vi "Open.vi"(8 "error in (no error)":errorcluster, 11 "MelsecTCP in":refnum<class "InovanceSerialModbusRtu.lvclass">) -> (0 "error out":errorcluster, 3 "MelsecTCP out":refnum<class "InovanceSerialModbusRtu.lvclass">)   [LabVIEW 2020, in "HslCommunication.lvlib" / "InovanceSerialModbusRtu.lvclass"]
uses:
  InovanceSerialModbusRtu.lvclass
  InovanceSerialModbusRtu.lvclass/InovanceSerialModbusRtu.ctl
  E:/Git/Libraries/develop/HslCommunication/_Dependenciecs/HslCommunication.dll
  _Dependenciecs/HslCommunication.dll
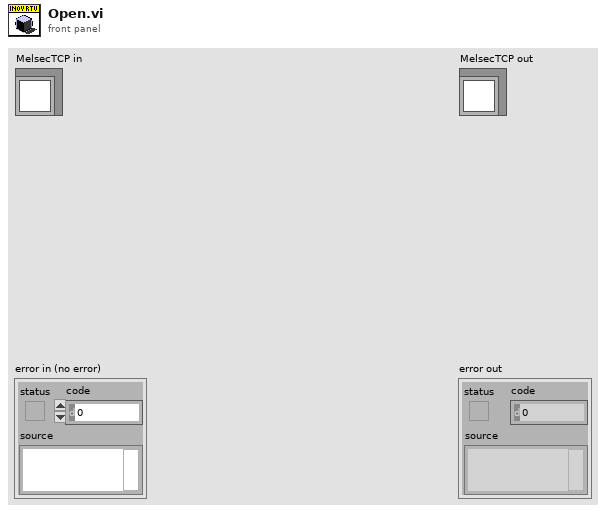
[diagram p1: front panel]
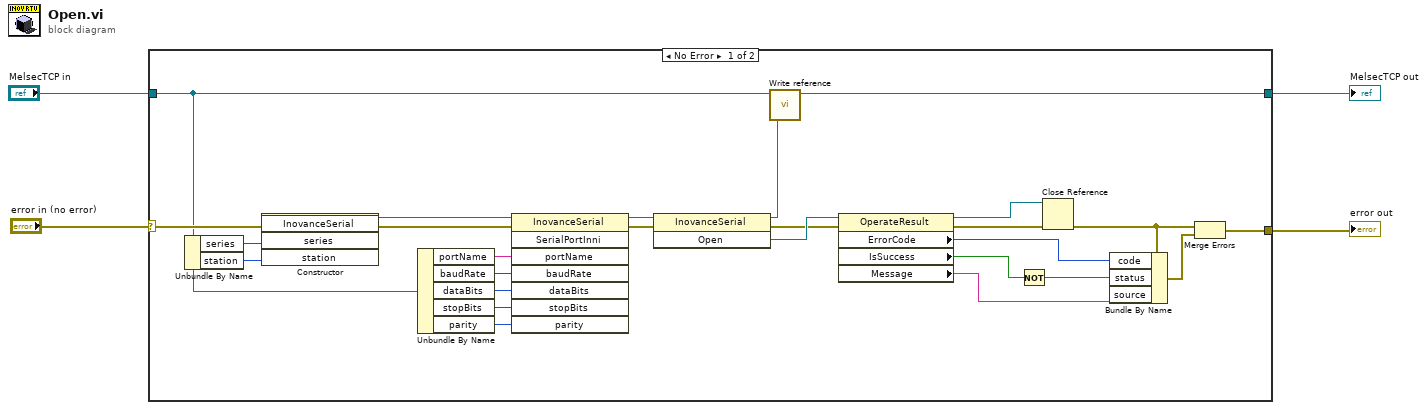
[diagram p0: block diagram]
diagram:
  n1 = case shown="No Error" "error in (no error)" {
    selector: "error in (no error)" -> [w18 w32]
    tunnel: "MelsecTCP in" -> [w13 w31]
    tunnel: [w6 w31] -> w1
    tunnel: [w25 w32] -> w2
    frame No Error {
      n2 = Unbundle By Name(w13) -> ("series"=w7:i32, "station"=w14:u8)
      n3 = constructor class="InovanceSerial"(error in=w18, "series"=w7, "station"=w14) -> (reference out=w22:refnum<k24>, error out=w21:errorcluster)  [unwired: 2 in, 3 out]
      n4 = Unbundle By Name(w13) -> ("portName"=w8:string, "baudRate"=w12:i32, "dataBits"=w11:i32, "stopBits"=w10:i32, "parity"=w9:i32)
      n5 = invoke class="InovanceSerial" method="SerialPortInni"(reference=w22, error in=w21, "portName"=w8, "baudRate"=w12, "dataBits"=w11, "stopBits"=w10, "parity"=w9) -> (reference out=w19:refnum<k24>, error out=w17:errorcluster)  [unwired: 1 in, 6 out]
      n6 = invoke class="InovanceSerial" method="Open"(reference=w19, error in=w17) -> (reference out=w5:refnum<k24>, error out=w15:errorcluster, "Open"=w16:refnum<k24>)  [unwired: 1 in]
      n7 = call-dynamic "Write reference.vi"("reference"=w5, "MelsecTCP in"=w13) -> ("MelsecTCP out"=w6:refnum<class "InovanceSerialModbusRtu.lvclass">)  [unwired: 8 in, 1 out]
      n8 = property class="OperateResult"(reference=w16, error in=w15) -> (reference out=w24:refnum<k24>, error out=w23:errorcluster, "ErrorCode"=w28:i32, "IsSuccess"=w20:bool, "Message"=w26:string)
      n9 = Not(x=w20) -> (.not. x?=w27:bool)
      n10 = Close Reference(reference=w24, error in (no error)=w23) -> (error out=w29:errorcluster)
      n11 = Bundle By Name(cluster=w29, "code"=w28, "status"=w27, "source"=w26) -> (w30:errorcluster)
      n12 = Merge Errors(w29, w30) -> (w25:errorcluster)
    }
    frame Error {
    }
  }
  "error out" <- w2
  "MelsecTCP out" <- w1
